vi "xscale.vi"() -> ()   [LabVIEW 2011]
panel:
  in  "Stop":bool
  in  "Range":dbl=10.0
  out "Waveform Chart":dbl(graph)
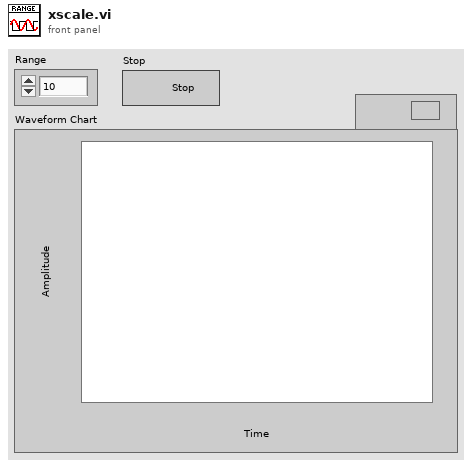
[diagram p1: front panel]
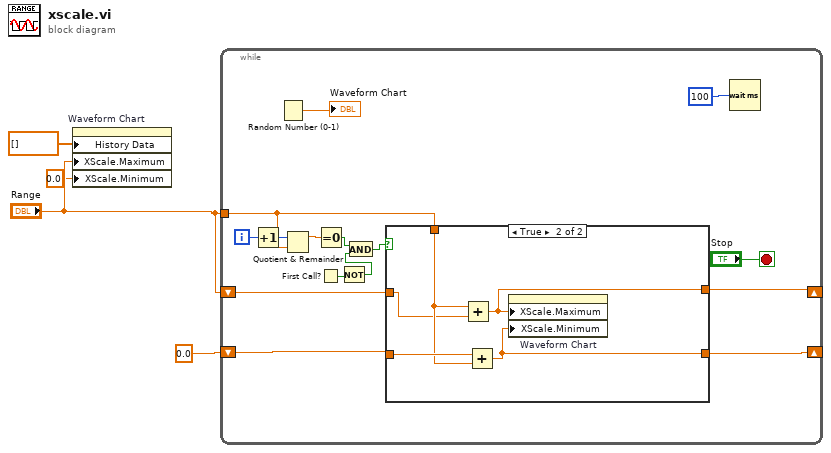
[diagram p0: block diagram]
diagram:
  n1 = property on="Waveform Chart" class="WFChart (strict)"("History Data"=dbl[] [], "XScale.Maximum"="Range", "XScale.Minimum"=0.0 ("X Scale.Range:Minimum")) -> ()  [unwired: 2 in, 2 out]
  n2 = while {
    shift-right: [w15] -> _
    shift-left: "Range" -> [w12]
    shift-right: [w13] -> _
    shift-left: 0.0 ("milliseconds to wait") -> [w14]
    tunnel: "Range" -> [w10]
    i -> [w11]
    stop <- "Stop" stop-if-true
    n3 = Increment(x=w11) -> (x+1=w5:i32)
    n4 = Random Number (0-1)() -> (number: 0 to 1=→"Waveform Chart":dbl)
    n5 = Quotient & Remainder(x=w5, y=w10) -> (x-y*floor(x/y)=w16:dbl)  [unwired: 1 out]
    n6 = Equal To 0?(x=w16) -> (x = 0?=w7:bool)
    n7 = First Call?() -> (First Call?: T/F=w9:bool)
    n8 = Not(x=w9) -> (.not. x?=w6:bool)
    n9 = And(x=w7, y=w6) -> (x .and. y?=w8:bool)
    n10 = case shown="True" w8 {
      tunnel: w10 -> [_ w23]
      tunnel: [w21 w26] -> w15
      tunnel: w14 -> [w20 w25]
      tunnel: [w20 w24] -> w13
      tunnel: w12 -> [w21 w22]
      frame False {
      }
      frame True {
        n11 = Add(x=w23, y=w22) -> (x+y=w26:dbl)
        n12 = Add(x=w25, y=w23) -> (x+y=w24:dbl)
        n13 = property on="Waveform Chart" class="WFChart (strict)"("XScale.Maximum"=w26, "XScale.Minimum"=w24) -> ()  [unwired: 2 in, 2 out]
      }
    }
    n14 = Wait (ms)(milliseconds to wait=u32 100) -> ()  [unwired: 1 out]
  }
